vi "Actor Core.vi"(8 "error in":errorcluster, 11 "VIStore in":refnum<class "VIStore.lvclass">) -> (0 "error out":errorcluster, 3 "Actor out":refnum<class "Actor.lvclass">)   [LabVIEW 2015, in "VI App Store.lvlib" / "VIStore.lvclass"]
doc: "(<B>Filename</B>: Actor Framework.lvlib:Actor.lvclass:Actor Core.vi)\n\nReceives messages to the actor, reacts to them, and initiates any error handling that may shut the actor down.\n\nDescendant classes may override this VI to append parallel tasks for the actor to complete while it handles messages. Overrides use the Call Parent Method node."
uses:
  VIStore.lvclass
  <vilib>/ActorFramework/Actor/Actor.lvclass
  Store UI/StoreUI Actor/StoreUI.lvclass
  VIStore.lvclass/VIStore.ctl
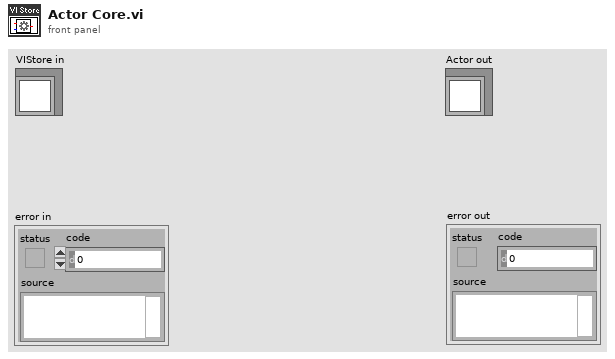
[diagram p1: front panel]
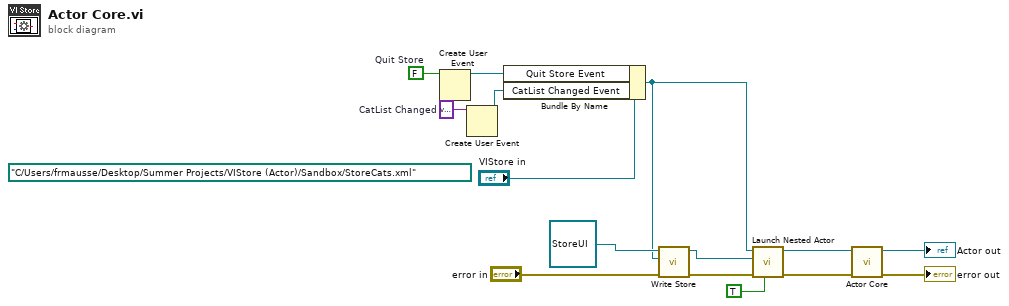
[diagram p0: block diagram]
diagram:
  w3 = variant  # CatList Changed
  w11 = FALSE  # Quit Store
  (unwired) path "C:/Users/frmausse/Desktop/Summer Projects/VIStore (Actor)/Sandbox/StoreCats.xml" ("Cats XML")
  n1 = Create User Event(user event datatype=w11) -> (user event=w10:refnum<user-event>)  [unwired: 1 in, 1 out]
  n2 = Create User Event(user event datatype=w3) -> (user event=w2:refnum<user-event>)  [unwired: 1 in, 1 out]
  n3 = Bundle By Name(cluster="VIStore in", "Quit Store Event"=w10, "CatList Changed Event"=w2) -> (w1:refnum<class "VIStore.lvclass">)
  n4 = call "Write Store.vi"("error in (no error)"="error in", "Store Actor"=w1, "StoreUI in"=refnum<class "StoreUI.lvclass"> refnum ("StoreUI.lvlib:StoreUI.lvclass")) -> ("error out"=w5:errorcluster, "StoreUI out"=w6:refnum<class "StoreUI.lvclass">)  [unwired: 7 in]
  n5 = call <vilib>:"Launch Nested Actor.vi"("Open Actor Core front panel? (F)"=TRUE, "error in (no error)"=w5, "Nested Actor"=w6, "Caller Actor in"=w1) -> ("error out"=w9:errorcluster, "Caller Actor out"=w12:refnum<class "VIStore.lvclass">)  [unwired: 5 in, 1 out]
  n6 = call-parent "Actor Core.vi"("error in"=w9, "Actor in"=w12) -> ("error out"=→"error out":errorcluster, "Actor out"=→"Actor out":refnum<class "Actor.lvclass">)  [unwired: 8 in]
